vi "Load Challenges.vi"(8 "error in (no error)":errorcluster, 11 "Challenge DB in":refnum<class "Challenge DB.lvclass">) -> (0 "error out":errorcluster, 3 "Challenge DB out":refnum<class "Challenge DB.lvclass">)   [LabVIEW 2020, in "Summer of LabVIEW.lvlib" / "Challenge DB.lvclass"]
uses:
  Challenge DB.lvclass
  Challenge DB.lvclass/Challenge DB.ctl
  Challenge/Challenge.lvclass
  <vilib>/drjdpowell/SQLite Library/SQL Statement/SQL Statement.lvclass/SQL Statement.ctl
  Challenge/Challenge Data.ctl
  <vilib>/drjdpowell/SQLite Library/SQL Statement/Column I64.vi
  <vilib>/drjdpowell/SQLite Library/SQL Statement/Error Message.vi
  <vilib>/drjdpowell/SQLite Library/SQL Statement/Column String.vi
  SQLite/SQLite.lvclass
  <vilib>/drjdpowell/SQLite Library/SQL Connection/Connection.lvclass
  <vilib>/drjdpowell/SQLite Library/SQL Statement/SQL Statement.lvclass
  <vilib>/IlluminatedG/lv-web-crypto/lv-json/JSON/JSON.lvlib
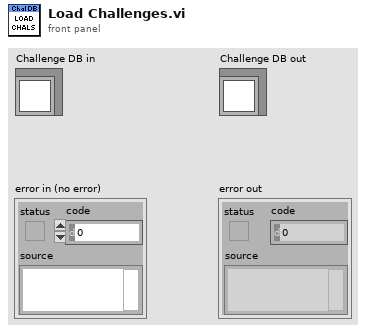
[diagram p1: front panel]
types:
  T1 = typedef "Summer of LabVIEW.lvlib/Challenge.lvclass/Challenge Data.ctl" = cluster{"ID":i64, "Name":string, "Description":string, "Download":string, "Instructions":string, "Start":timestamp, "End":timestamp}
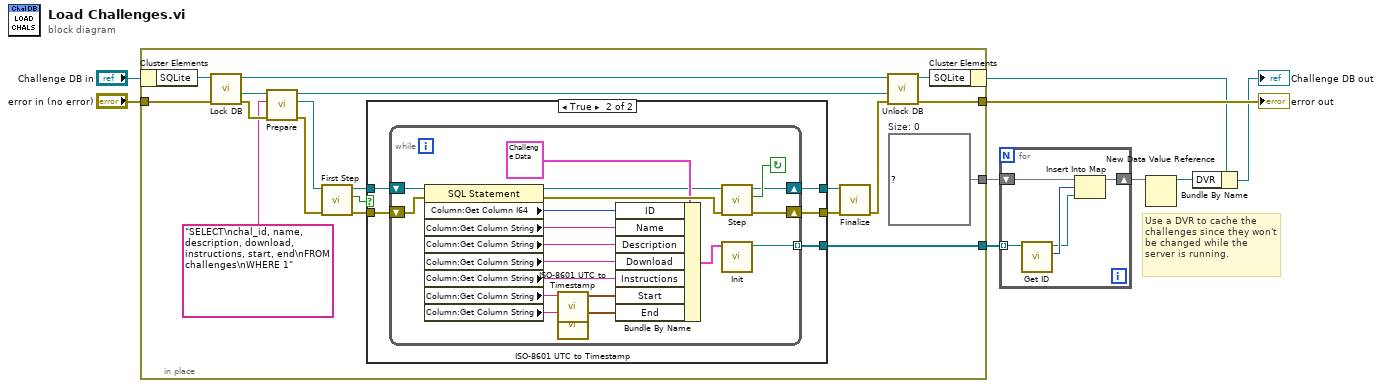
[diagram p0: block diagram]
diagram:
  # "Use a DVR to cache the challenges since they won't be changed while the server is running."
  n1 = in-place {
    in-place-border: "error in (no error)" -> [w27]
    in-place-border: [w13] -> w7
    in-place-border: [w11] -> w6
    in-place-border: [w10] -> w5
    w10 = map{i64, refnum<class "Challenge.lvclass">} {}  # Size: 0
    n2 = in-place-cluster #1("Challenge DB in") -> ("SQLite"=w28:refnum<class "SQLite.lvclass">)
    n3 = call "Lock DB.vi"("error in (no error)"=w27, "SQLite in"=w28) -> ("error out"=w25:errorcluster, "SQLite DB"=w26:refnum<class "Connection.lvclass">, "SQLite out"=w17:refnum<class "SQLite.lvclass">)  [unwired: 6 in, 1 out]
    n4 = call <vilib>:"Prepare.vi"("error in (no error)"=w25, "SQL"="SELECT\nchal_id, name, description, download, instructions, start, end\nFROM challenges\nWHERE 1", "SQLite Connection in"=w26) -> ("error out"=w22:errorcluster, "SQL Statement"=w24:refnum<class "SQL Statement.lvclass">, "SQLite Connection"=w15:refnum<class "Connection.lvclass">)  [unwired: 4 in, 2 out]
    n5 = call <vilib>:"First Step.vi"("error in (no error)"=w22, "SQL Statement in"=w24) -> ("error out"=w21:errorcluster, "Row returned"=w23:bool, "SQL Statement"=w20:refnum<class "SQL Statement.lvclass">)  [unwired: 7 in]
    n6 = case shown="True" w23 {
      tunnel: w21 -> [w29 w34]
      tunnel: w20 -> [w30 w35]
      tunnel: [w30 w32] -> w19
      tunnel: [w29 w31] -> w18
      tunnel: [_ w33] -> w11
      frame False {
      }
      frame True {
        n7 = while {
          shift-right: [w42] -> w32
          shift-left: w35 -> [w53]
          shift-right: [w41] -> w31
          shift-left: w34 -> [w52]
          tunnel: [w40] -> w33 mode=indexing
          stop <- w43 continue-if-true
          n8 = property on="Extract Column Data" class="SQL Statement"(reference=w53, error in=w52) -> (reference out=w44:refnum<class "SQL Statement.lvclass">, error out=w54:errorcluster, "Column:Get Column I64"=w50:i64, "Column:Get Column String"=w49:string, "Column:Get Column String"=w46:string, "Column:Get Column String"=w47:string, "Column:Get Column String"=w48:string, "Column:Get Column String"=w39:string, "Column:Get Column String"=w38:string)
          n9 = call <vilib>:"ISO-8601 UTC to Timestamp.vi"("ISO-8601"=w39) -> ("time stamp"=w37:timestamp)  [unwired: 9 in, 1 out]
          n10 = call <vilib>:"ISO-8601 UTC to Timestamp.vi"("ISO-8601"=w38) -> ("time stamp"=w36:timestamp)  [unwired: 9 in, 1 out]
          n11 = Bundle By Name(cluster=T1 {"ID"=0, "Name"="", "Description"="", "Download"="", "Instructions"="", "Start"=timestamp(0 s since 1904-01-01), "End"=timestamp(0 s since 1904-01-01)} ("Challenge Data"), "ID"=w50, "Name"=w49, "Description"=w46, "Download"=w47, "Instructions"=w48, "Start"=w37, "End"=w36) -> (w45:T1)
          n12 = call <vilib>:"Step.vi"("error in (no error)"=w54, "SQL Statement in"=w44) -> ("error out"=w41:errorcluster, "Row returned"=w43:bool, "SQL Statement"=w42:refnum<class "SQL Statement.lvclass">)  [unwired: 7 in]
          n13 = call "Init.vi"("Challenge Data"=w45) -> ("Challenge out"=w40:refnum<class "Challenge.lvclass">)  [unwired: 9 in, 1 out]
        }
      }
    }
    n14 = call <vilib>:"Finalize.vi"("error in (no error)"=w18, "SQL Statement in"=w19) -> ("error out"=w16:errorcluster)  [unwired: 9 in]
    n15 = call "Unlock DB.vi"("error in (no error)"=w16, "SQLite DB"=w15, "SQLite in"=w17) -> ("error out"=w13:errorcluster, "SQLite out"=w14:refnum<class "SQLite.lvclass">)  [unwired: 7 in]
    n16 = in-place-cluster #1("SQLite"=w14) -> (w4:refnum<class "Challenge DB.lvclass">)
  }
  "error out" <- w7
  n17 = for {
    tunnel: w6 -> [w59] mode=indexing
    shift-right: [w55] -> w3
    shift-left: w5 -> [w58]
    n18 = call "Get ID.vi"("Challenge in"=w59) -> ("ID"=w57:i64, "Challenge out"=w56:refnum<class "Challenge.lvclass">)  [unwired: 9 in]
    n19 = Insert Into Map(map in=w58, key=w57, value=w56) -> (map out=w55:map{i64, refnum<class "Challenge.lvclass">})  [unwired: 2 out]
  }
  n20 = New Data Value Reference(data value=w3) -> (data value reference=w2:refnum<data-value>)  [unwired: 1 in, 1 out]
  n21 = Bundle By Name(cluster=w4, "DVR"=w2) -> (→"Challenge DB out":refnum<class "Challenge DB.lvclass">)
